vi "Get Projects.vi"(0 "Ring refnum":refnum<vi>, 11 "error in (no error)":errorcluster) -> (4 "Project:Projects[]":refnum<vi>[](array[refnum]), 15 "error out":errorcluster)   [LabVIEW 2015, in "UIM.lvclass"]
uses:
  UIM.lvclass
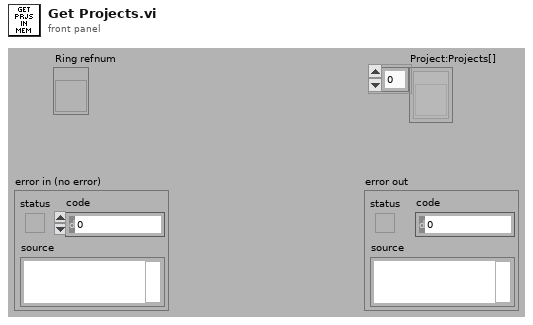
[diagram p1: front panel]
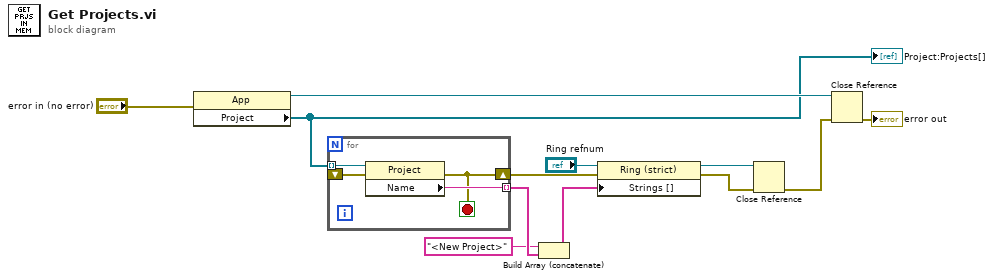
[diagram p0: block diagram]
diagram:
  n1 = property class="App"(error in="error in (no error)") -> (reference out=w12:refnum<vi>, "Project"=w11:refnum<vi>[])  [unwired: 1 in, 1 out]
  "Project:Projects[]" <- w11
  n2 = for {
    tunnel: w11 -> [w16] mode=indexing
    shift-right: [w13] -> w6
    shift-left: _ -> [w15]
    tunnel: [w14] -> w7 mode=indexing
    stop <- w13 stop-if-true
    n3 = property class="Project"(reference=w16, error in=w15) -> (error out=w13:errorcluster, "Name"=w14:string)  [unwired: 1 out]
  }
  n4 = Build Array (concatenate)("<New Project>", w7) -> (w2:string[])
  n5 = property class="Ring (strict)"(reference="Ring refnum", error in=w6, "Strings []"=w2) -> (reference out=w10:refnum<vi>, error out=w9:errorcluster)
  n6 = Close Reference(reference=w10, error in (no error)=w9) -> (error out=w3:errorcluster)
  n7 = Close Reference(reference=w12, error in (no error)=w3) -> (error out=→"error out":errorcluster)
